vi "HeaderBis.vi"(0 "UUTHeader":string, 1 "UA":string, 2 "POWER SN":string, 3 "Revision Param":string, 5 "P/N UUT":string, 7 "DSP SN":string, 9 "Driver S/N":string, 11 "error in":errorcluster, 12 "VR":string, 13 "Oper.":string, 14 "Tester Software Ver":string) -> (4 "table header":string, 6 "Array":string[][](array[string]), 15 "error out":errorcluster)   [LabVIEW 2017]
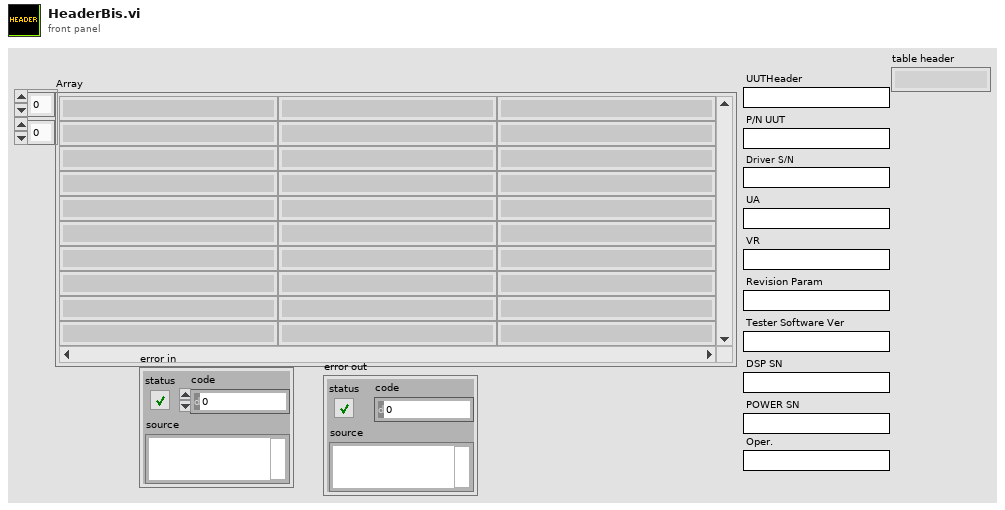
[diagram p1: front panel]
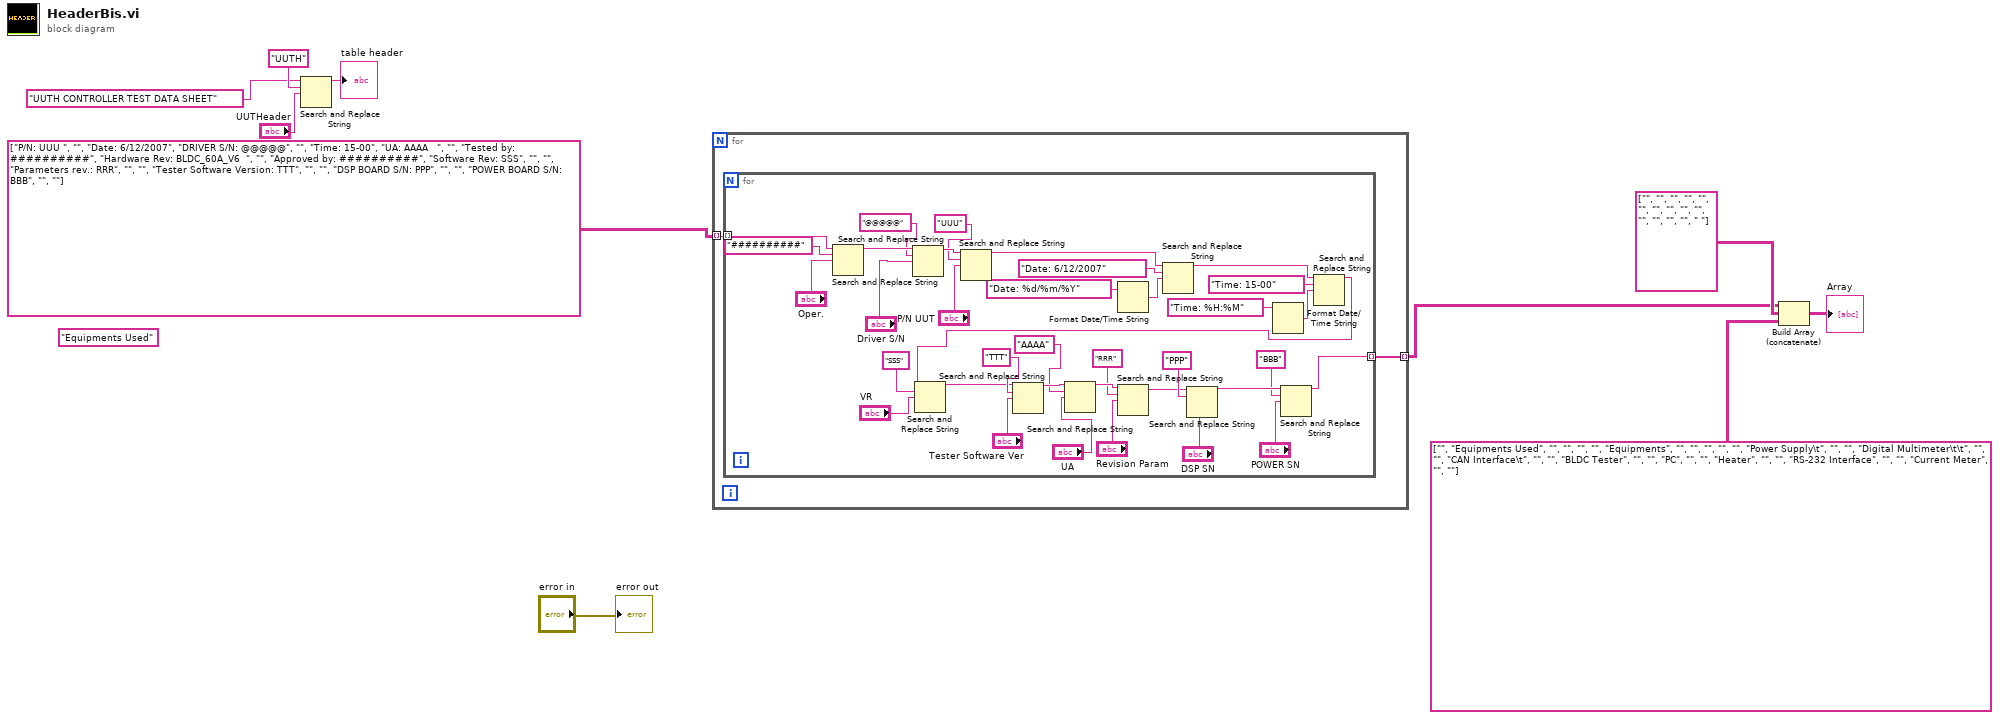
[diagram p0: block diagram]
diagram:
  (unwired) "Equipments Used"
  n1 = Search and Replace String(input string="UUTH CONTROLLER TEST DATA SHEET", search string="UUTH", replace string="UUTHeader") -> (result string=→"table header":string)  [unwired: 5 in, 3 out]
  n2 = for {
    tunnel: string[][] [["P/N: UUU ", "", "Date: 6/12/2007"], ["DRIVER S/N: @@@@@", "", "Time: 15-00"], ["UA: AAAA   ", "", "Tested by: ##########"], ["Hardware Rev: BLDC_60A_V6  ", "", "Approved by: ##########"], ["Software Rev: SSS", "", ""], ["Parameters rev.: RRR", "", ""], ["Tester Software Version: TTT", "", ""], ["DSP BOARD S/N: PPP", "", ""], ["POWER BOARD S/N: BBB", "", ""]] -> [w12] mode=indexing
    tunnel: [w11] -> w3 mode=indexing
    n3 = for {
      tunnel: w12 -> [w21] mode=indexing
      tunnel: [w14] -> w11 mode=indexing
      n4 = Search and Replace String(input string=w21, search string="##########" ("source"), replace string="Oper.") -> (result string=w34:string)  [unwired: 5 in, 3 out]
      n5 = Search and Replace String(input string=w34, search string="@@@@@" ("source"), replace string="Driver S/N") -> (result string=w36:string)  [unwired: 5 in, 3 out]
      n6 = Search and Replace String(input string=w36, search string="UUU" ("source"), replace string="P/N UUT") -> (result string=w35:string)  [unwired: 5 in, 3 out]
      n7 = Format Date/Time String(time format string (%c)="Date: %d/%m/%Y") -> (date/time string=w33:string)  [unwired: 2 in]
      n8 = Search and Replace String(input string=w35, search string="Date: 6/12/2007" ("time format string (%c)"), replace string=w33) -> (result string=w44:string)  [unwired: 5 in, 3 out]
      n9 = Format Date/Time String(time format string (%c)="Time: %H:%M") -> (date/time string=w46:string)  [unwired: 2 in]
      n10 = Search and Replace String(input string=w44, search string="Time: 15-00", replace string=w46) -> (result string=w45:string)  [unwired: 5 in, 3 out]
      n11 = Search and Replace String(input string=w45, search string="SSS", replace string="VR") -> (result string=w13:string)  [unwired: 5 in, 3 out]
      n12 = Search and Replace String(input string=w13, search string="TTT", replace string="Tester Software Ver") -> (result string=w42:string)  [unwired: 5 in, 3 out]
      n13 = Search and Replace String(input string=w42, search string="AAAA", replace string="UA") -> (result string=w48:string)  [unwired: 5 in, 3 out]
      n14 = Search and Replace String(input string=w48, search string="RRR", replace string="Revision Param") -> (result string=w18:string)  [unwired: 5 in, 3 out]
      n15 = Search and Replace String(input string=w18, search string="PPP", replace string="DSP SN") -> (result string=w17:string)  [unwired: 5 in, 3 out]
      n16 = Search and Replace String(input string=w17, search string="BBB", replace string="POWER SN") -> (result string=w14:string)  [unwired: 5 in, 3 out]
    }
  }
  n17 = Build Array (concatenate)(w3, string[][] [["", "", ""], ["", "", ""], ["", "", ""], ["", "", ""], ["", "", " "]], string[][] [["", "Equipments Used", ""], ["", "", ""], ["Equipments", "", ""], ["", "", ""], ["Power Supply\t", "", ""], ["Digital Multimeter\t\t", "", ""], ["CAN Interface\t", "", ""], ["BLDC Tester", "", ""], ["PC", "", ""], ["Heater", "", ""], ["RS-232 Interface", "", ""], ["Current Meter", "", ""]]) -> (→"Array":string[][])
  "error out" <- "error in"
